vi "Get Message Broker.vi"(8 "error in (no error)":errorcluster, 11 "Message Broker Interface Ref in":refnum<class "Message Broker Interface Ref.lvclass">) -> (0 "error out":errorcluster, 2 "Broker":refnum<data-value>, 3 "Message Broker Interface Ref out":refnum<class "Message Broker Interface Ref.lvclass">)   [LabVIEW 2016, in "Stream Mediator.lvlib" / "Message Broker Interface Ref.lvclass"]
uses:
  <userlib>/Composed Systems/Stream/Mediator/Classes/Message Broker Interface Ref/Message Broker Interface Ref.lvclass
  <userlib>/Composed Systems/Stream/Mediator/Classes/Message Broker/Message Broker.lvclass
  <userlib>/Composed Systems/Stream/Mediator/Classes/Message Broker Interface Ref/Message Broker Interface Ref.lvclass/Message Broker Interface Ref.ctl
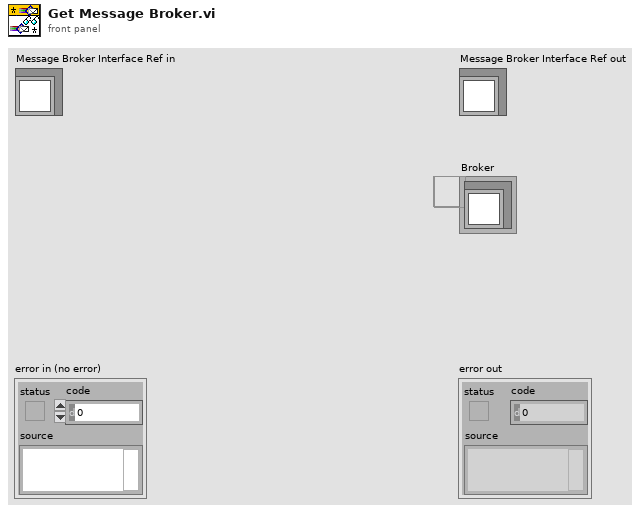
[diagram p1: front panel]
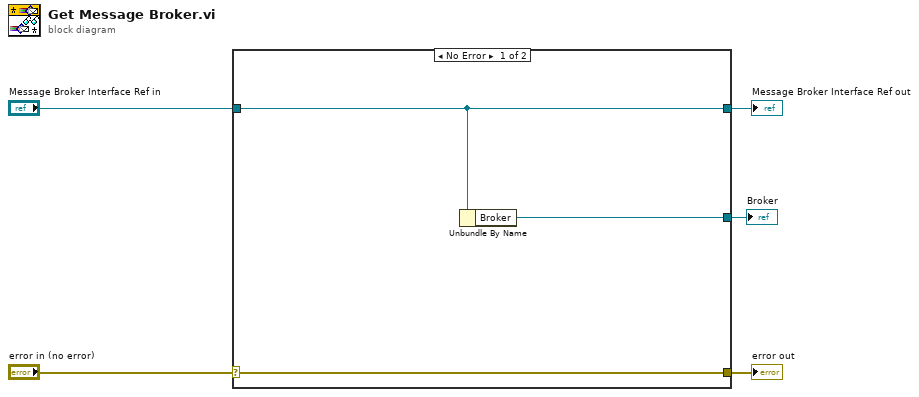
[diagram p0: block diagram]
diagram:
  n1 = case shown="No Error" "error in (no error)" {
    selector: "error in (no error)" -> [w8 w10]
    tunnel: [w8 w10] -> w4
    tunnel: [w7 w9] -> w2
    tunnel: "Message Broker Interface Ref in" -> [w7 w9]
    tunnel: [w6 _] -> w1
    frame No Error {
      n2 = Unbundle By Name(w7) -> ("Broker"=w6:refnum<data-value>)
    }
    frame Error {
    }
  }
  "error out" <- w4
  "Message Broker Interface Ref out" <- w2
  "Broker" <- w1
